vi "Supported Smart Syntax Representation.vi"(0 "String Operations in":refnum<class "String Operations.lvclass">, 11 "error in (no error)":errorcluster) -> (4 "String Operations out":refnum<class "String Operations.lvclass">, 6 "Smart Syntax Representation List":string[](array[string]), 15 "error out":errorcluster)   [LabVIEW 2016, in "String Operations.lvclass"]
uses:
  String Operations.lvclass
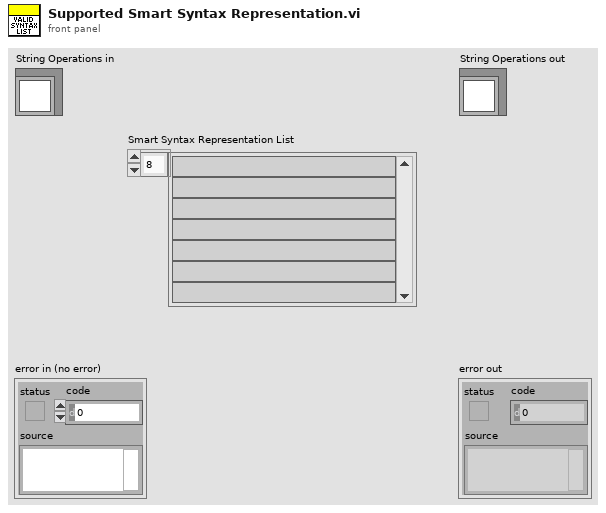
[diagram p1: front panel]
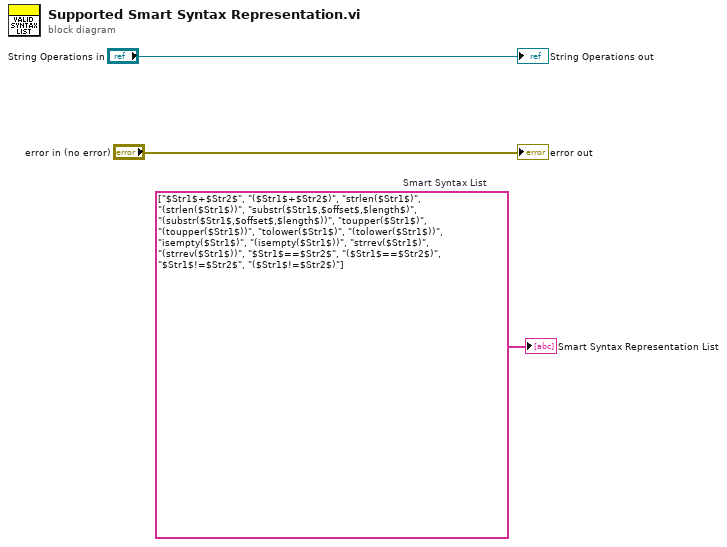
[diagram p0: block diagram]
diagram:
  w1 = string[] ["$Str1$+$Str2$", "($Str1$+$Str2$)", "strlen($Str1$)", "(strlen($Str1$))", "substr($Str1$,$offset$,$length$)", "(substr($Str1$,$offset$,$length$))", "toupper($Str1$)", "(toupper($Str1$))", "tolower($Str1$)", "(tolower($Str1$))", "isempty($Str1$)", "(isempty($Str1$))", "strrev($Str1$)", "(strrev($Str1$))", "$Str1$==$Str2$", "($Str1$==$Str2$)", "$Str1$!=$Str2$", "($Str1$!=$Str2$)"]  # Smart Syntax List
  "error out" <- "error in (no error)"
  "String Operations out" <- "String Operations in"
  "Smart Syntax Representation List" <- w1
